vi "UnloadInterface.vi"(0 "Interface en entrée":refnum<class "Interface.lvclass"> caption="DNL_LabVIEW Object in", 11 "error in (no error)":errorcluster caption="entrée d'erreur (pas d'erreur)") -> (4 "Interface en sortie":refnum<class "Interface.lvclass"> caption="DNL_LabVIEW Object out", 6 "Graph_FA":refnum<vi>[](array[refnum]), 8 "PanRef":refnum<vi>, 10 "ListBoxRef":refnum<vi>, 14 "BaseDataPath":path, 15 "error out":errorcluster caption="sortie d'erreur")   [LabVIEW 2019, in "Interface.lvclass"]
uses:
  Interface.lvclass
  Interface.lvclass/Interface.ctl
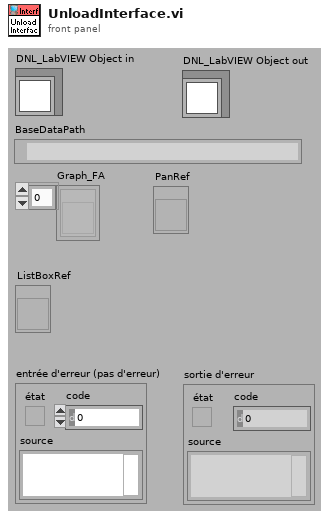
[diagram p1: front panel]
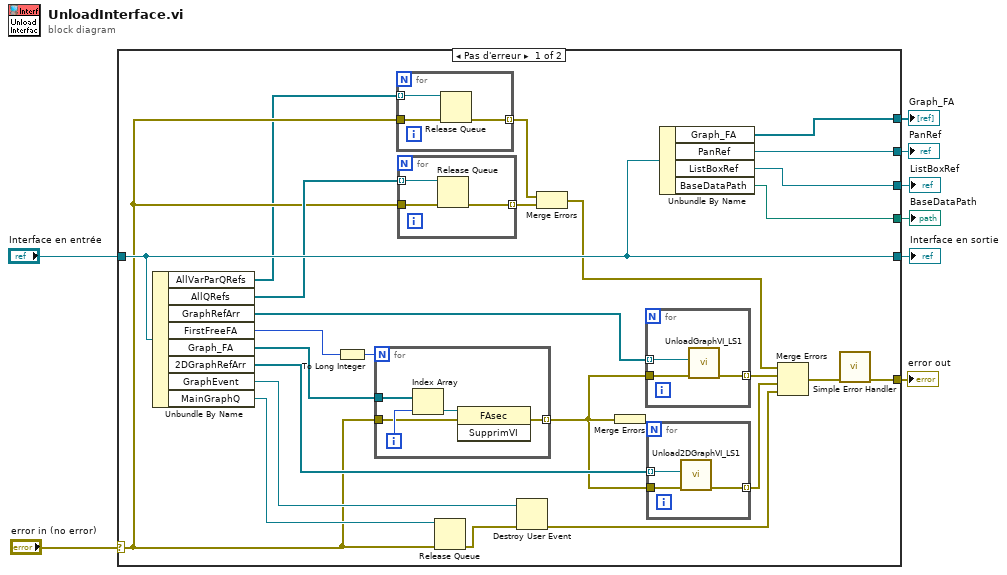
[diagram p0: block diagram]
diagram:
  n1 = case shown="Pas d'erreur" "error in (no error)" {
    selector: "error in (no error)" -> [w12 w53]
    tunnel: [w20 w53] -> w7
    tunnel: [w29 w52] -> w5
    tunnel: "Interface en entrée" -> [w29 w52]
    tunnel: [w28 _] -> w4
    tunnel: [w27 _] -> w3
    tunnel: [w26 _] -> w2
    tunnel: [w25 _] -> w1
    frame No Error {
      n2 = Unbundle By Name(w29) -> ("AllVarParQRefs"=w10:refnum<queue>[], "AllQRefs"=w24:refnum<queue>[], "GraphRefArr"=w30:refnum<vi>[], "FirstFreeFA"=w31:u8, "Graph_FA"=w32:refnum<vi>[], "2DGraphRefArr"=w19:refnum<vi>[], "GraphEvent"=w15:refnum<user-event>, "MainGraphQ"=w16:refnum<queue>)
      n3 = To Long Integer(number=w31) -> (32bit integer=w33:i32)
      n4 = for {
        N: w33 -> [_]
        tunnel: w32 -> [w45]
        tunnel: w12 -> [w42]
        tunnel: [w41] -> w21 mode=indexing
        i -> [w44]
        n5 = Index Array(array=w45, index=w44) -> (element=w43:refnum<vi>)
        n6 = invoke class="FAsec" method="SupprimVI"(reference=w43, error in=w42) -> (error out=w41:errorcluster)  [unwired: 1 in, 2 out]
      }
      n7 = for {
        tunnel: w12 -> [w35]
        tunnel: [w37] -> w11 mode=indexing
        tunnel: w10 -> [w36] mode=indexing
        n8 = Release Queue(queue=w36, error in (no error)=w35) -> (error out=w37:errorcluster)  [unwired: 1 in, 2 out]
      }
      n9 = for {
        tunnel: w24 -> [w38] mode=indexing
        tunnel: w12 -> [w39]
        tunnel: [w40] -> w22 mode=indexing
        n10 = Release Queue(queue=w38, error in (no error)=w39) -> (error out=w40:errorcluster)  [unwired: 1 in, 2 out]
      }
      n11 = Release Queue(queue=w16, error in (no error)=w12) -> (error out=w14:errorcluster)  [unwired: 1 in, 2 out]
      n12 = Destroy User Event(user event=w15, error in=w14) -> (error out=w13:errorcluster)
      n13 = Merge Errors(w11, w22) -> (w9:errorcluster)
      n14 = Merge Errors(w21) -> (w18:errorcluster)
      n15 = for {
        tunnel: w30 -> [w51] mode=indexing
        tunnel: w18 -> [w49]
        tunnel: [w50] -> w34 mode=indexing
        n16 = call "UnloadGraphVI_LS1.vi"("ErrorIn(No Error)"=w49, "GraphRef"=w51) -> ("sortie d'erreur"=w50:errorcluster)  [unwired: 9 in]
      }
      n17 = for {
        tunnel: w19 -> [w48] mode=indexing
        tunnel: w18 -> [w47]
        tunnel: [w46] -> w17 mode=indexing
        n18 = call "Unload2DGraphVI_LS1.vi"("ErrorIn(No Error)"=w47, "GraphRef"=w48) -> ("sortie d'erreur"=w46:errorcluster)  [unwired: 9 in]
      }
      n19 = Unbundle By Name(w29) -> ("Graph_FA"=w28:refnum<vi>[], "PanRef"=w27:refnum<vi>, "ListBoxRef"=w26:refnum<vi>, "BaseDataPath"=w25:path)
      n20 = Merge Errors(w9, w34, w17, w13) -> (w23:errorcluster)
      n21 = call <vilib>:"Simple Error Handler.vi"("error in (no error)"=w23) -> ("error out"=w20:errorcluster)  [unwired: 4 in, 4 out]
    }
    frame Error {
    }
  }
  "error out" <- w7
  "Interface en sortie" <- w5
  "Graph_FA" <- w4
  "PanRef" <- w3
  "ListBoxRef" <- w2
  "BaseDataPath" <- w1
